vi "VCS Get Object_String.vi"(0 "axis in":cluster{"keyHandle":u32, "nodeId":u16}={"keyHandle"=0, "nodeId"=1}, 5 "object in":T1 {"object subIndex" format="%x"; "object index" format="%x"}, 11 "error in (no error)":errorcluster) -> (4 "axis out":cluster{"keyHandle":u32, "nodeId":u16}={"keyHandle"=0, "nodeId"=1}, 10 "text":string, 15 "error out":errorcluster)   [LabVIEW 2010]
doc: "<B>VCS GetObject</B> reads an UINT32 object value at the given index and sub index from object dictionary."
uses:
  Resources/EposCmd.dll
  Resources/EposCmd64.dll
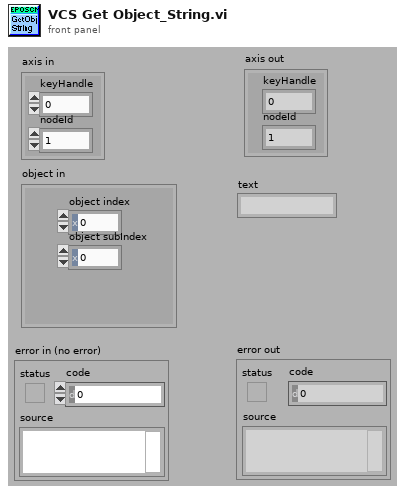
[diagram p1: front panel]
types:
  T1 = cluster{"object index":u16, "object subIndex":u8}
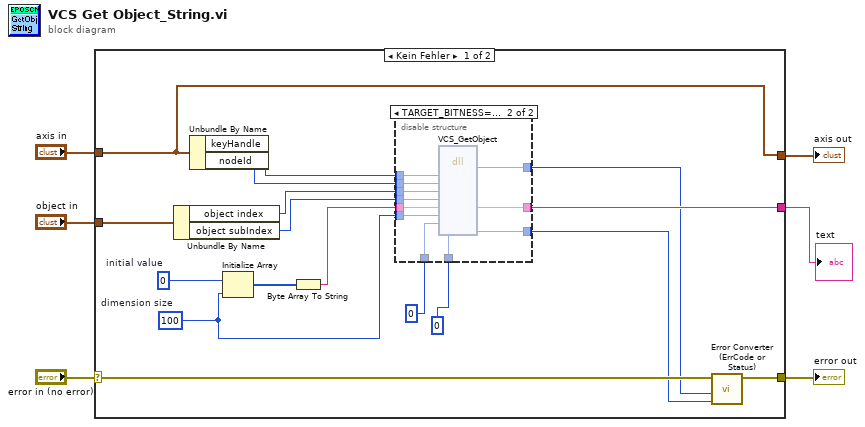
[diagram p0: block diagram]
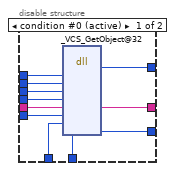
[diagram p2: hidden frame]
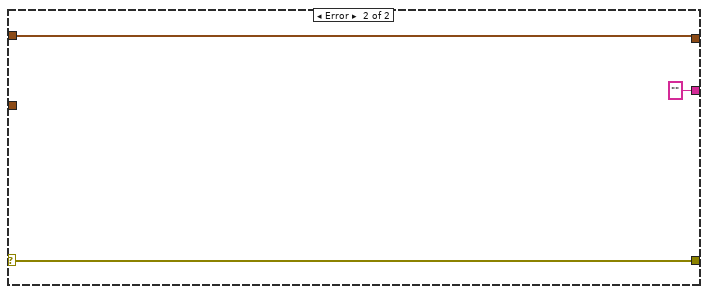
[diagram p3: hidden frame]
diagram:
  n1 = case shown="Kein Fehler" "error in (no error)" {
    selector: "error in (no error)" -> [w14 w48]
    tunnel: [w15 w48] -> w5
    tunnel: "axis in" -> [w18 w47]
    tunnel: "object in" -> [w19 _]
    tunnel: [w18 w47] -> w2
    tunnel: [w9 "" ("pData")] -> w1
    frame No Error {
      w10 = u32 100  # dimension size
      w12 = u32 0  # initial value
      n2 = Unbundle By Name(w19) -> ("object index"=w20:u16, "object subIndex"=w21:u8)
      n3 = Unbundle By Name(w18) -> ("keyHandle"=w23:u32, "nodeId"=w22:u16)
      n4 = Initialize Array(w12, w10) -> (w11:u32[])
      n5 = Byte Array To String(unsigned byte array=w11) -> (string=w13:string)
      n6 = disable-structure shown="TARGET_BITNESS==64" {
        disable-tunnel: w23 -> [w34 w45]
        disable-tunnel: w22 -> [w33 w44]
        disable-tunnel: w21 -> [w32 w43]
        disable-tunnel: w20 -> [w31 w42]
        disable-tunnel: u32 0 ("pNbOfBytesRead") -> [w30 w41]
        disable-tunnel: u32 0 ("pErrorCode") -> [w29 w40]
        disable-tunnel: w13 -> [w28 w39]
        disable-tunnel: w10 -> [w27 w38]
        disable-tunnel: [w26 w37] -> w9
        disable-tunnel: [w25 w36] -> w8
        disable-tunnel: [w24 w35] -> w7
        frame condition #0 (active) {
          n7 = dll-call lib="C:/Temp/maxon EPOS/Resources/EposCmd.*" fn="_VCS_GetObject@32"("KeyHandle"=w34, "NodeId"=w33, "ObjectIndex"=w31, "ObjectSubIndex"=w32, "pData"=w28, "NbOfBytesToRead"=w27, "pNbOfBytesRead"=w30, "pErrorCode"=w29) -> (w25:i32, "pData"=w26:string, "pErrorCode"=w24:u32)  [unwired: 9 in, 2 out]
        }
        frame condition #1 {
          n8 = dll-call lib="C:/setup/Resources/EposCmd64.*" fn="VCS_GetObject" ("EposCmd.dll:_VCS_GetObject@32")("KeyHandle"=w45, "NodeId"=w44, "ObjectIndex"=w42, "ObjectSubIndex"=w43, "pData"=w39, "NbOfBytesToRead"=w38, "pNbOfBytesRead"=w41, "pErrorCode"=w40) -> ("Rückgabetyp"=w36:i32, "pData"=w37:string, "pErrorCode"=w35:u32)  [unwired: 9 in, 2 out]
        }
      }
      n9 = call "Error Converter (ErrCode or Status).vi"("error code"=w7, "return type"=w8, "error in (no error)"=w14) -> ("error out"=w15:errorcluster)  [unwired: 7 in]
    }
    frame Error {
    }
  }
  "error out" <- w5
  "axis out" <- w2
  "text" <- w1
